vi "Configure Output.vi"(0 "VISA resource name":refnum<visa-resource-name>, 1 "Auto Output-Off (F: Disable)":bool, 2 "Auto Output-On (T: Enable)":bool=TRUE, 3 "Enable High Capacitance (F: Disable)":bool, 5 "Channel (0: Channel 1)":i32(ring) items=["Channel 1", "Channel 2"], 9 "Low Terminal State (1: Ground)":i32(ring)=1 items=["Float", "Ground"], 11 "error in (no error)":errorcluster, 12 "Output-Off Status (2: Normal)":i32(ring)=2 items=["Zero", "HIZ", "Normal"]) -> (4 "VISA resource name out":refnum<visa-resource-name>, 15 "error out":errorcluster)   [LabVIEW 2026, in "Agilent B2900 Series.lvlib"]
doc: "Change settings for channel output."
uses:
  Agilent B2900 Series.lvlib
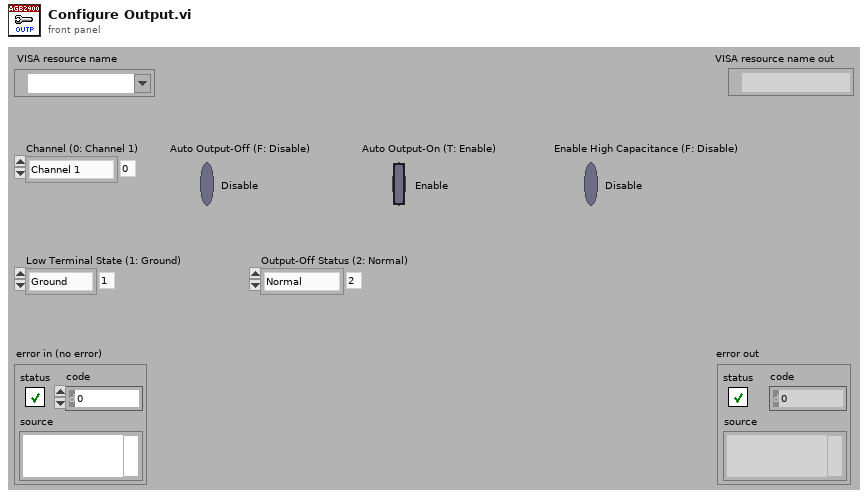
[diagram p1: front panel]
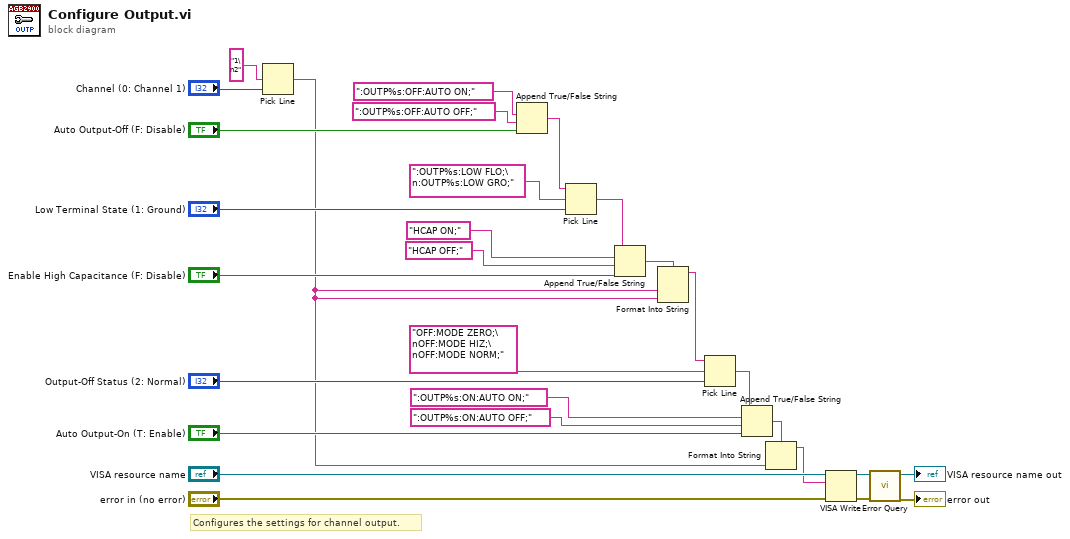
[diagram p0: block diagram]
diagram:
  # "Configures the settings for channel output."
  n1 = Pick Line(multi-line string="1\n2" ("string (\"\")"), line index="Channel (0: Channel 1)") -> (output string=w1:string)  [unwired: 1 in]
  n2 = Append True/False String(1:"Auto Output-Off (F: Disable)", 2:":OUTP%s:OFF:AUTO OFF;", 3:":OUTP%s:OFF:AUTO ON;") -> (0:w3:string)  [unwired: 1 in]
  n3 = Pick Line(string ("")=w3, multi-line string=":OUTP%s:LOW FLO;\n:OUTP%s:LOW GRO;", line index="Low Terminal State (1: Ground)") -> (output string=w21:string)
  n4 = Append True/False String(1:"Enable High Capacitance (F: Disable)", 2:"HCAP OFF;", 3:"HCAP ON;", 4:w21) -> (0:w2:string)
  n5 = Format Into String(format string=w2, w1, w1) -> (resulting string=w11:string)  [unwired: 2 in, 1 out]
  n6 = Pick Line(string ("")=w11, multi-line string="OFF:MODE ZERO;\nOFF:MODE HIZ;\nOFF:MODE NORM;", line index="Output-Off Status (2: Normal)") -> (output string=w27:string)
  n7 = Append True/False String(1:"Auto Output-On (T: Enable)", 2:":OUTP%s:ON:AUTO OFF;", 3:":OUTP%s:ON:AUTO ON;", 4:w27) -> (0:w9:string)
  n8 = Format Into String(format string=w9, w1) -> (resulting string=w10:string)  [unwired: 2 in, 1 out]
  n9 = VISA Write(VISA resource name="VISA resource name", write buffer=w10, error in (no error)="error in (no error)") -> (VISA resource name out=w15:refnum<visa-resource-name>, error out=w14:errorcluster)  [unwired: 1 out]
  n10 = call "Error Query.vi"("error in (no error)"=w14, "VISA resource name"=w15) -> ("error out"=→"error out":errorcluster, "VISA resource name out"=→"VISA resource name out":refnum<visa-resource-name>)  [unwired: 6 in, 2 out]
